vi "Test Func Mask.vi"() -> ()   [LabVIEW 2016]
uses:
  <vilib>/measure/mamon.llb/Create Continuous Mask using Formula.vi
  <vilib>/measure/mamon.llb/Limit Testing Time.vi
  <vilib>/measure/NI_MAPro.lvlib
  <vilib>/measure/NI_MABase.lvlib
panel:
  out "Limit":cluster{"x0":dbl, "dx":dbl, "Y":dbl[]} {"Y" format="%.2p"; "dx" format="%.2p"; "x0" format="%.2p"}
  out "Waveform Graph 3":waveform(dbl)[](graph)
  in  "stop":bool
  out "Waveform Graph":waveform(dbl)(graph)
  in  "signal type":T1(ring)
  in  "frequency":dbl=10.0 format="%0.2p"
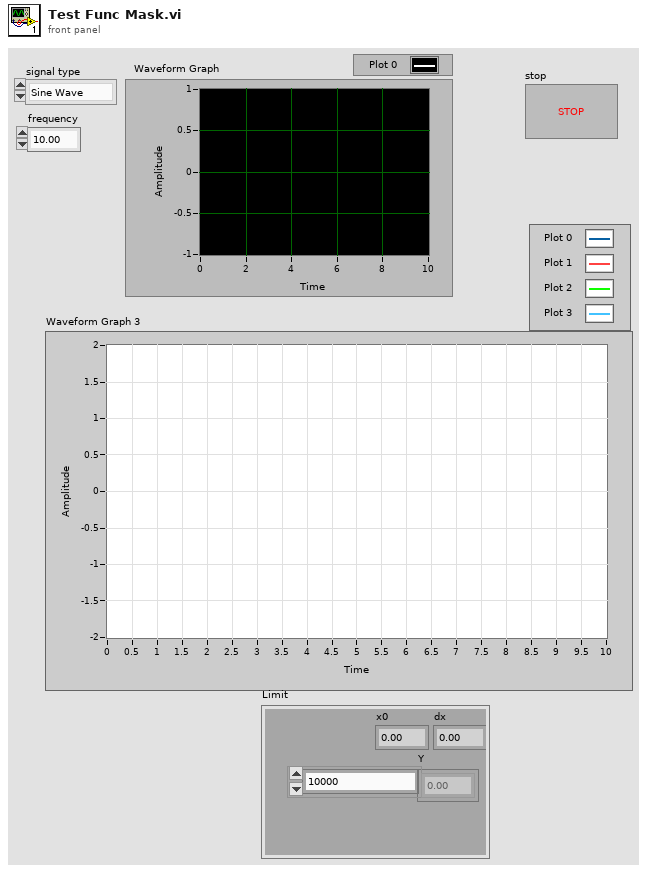
[diagram p1: front panel]
types:
  T1 = enum16{"Sine Wave", "Triangle Wave", "Square Wave", "Sawtooth Wave"}
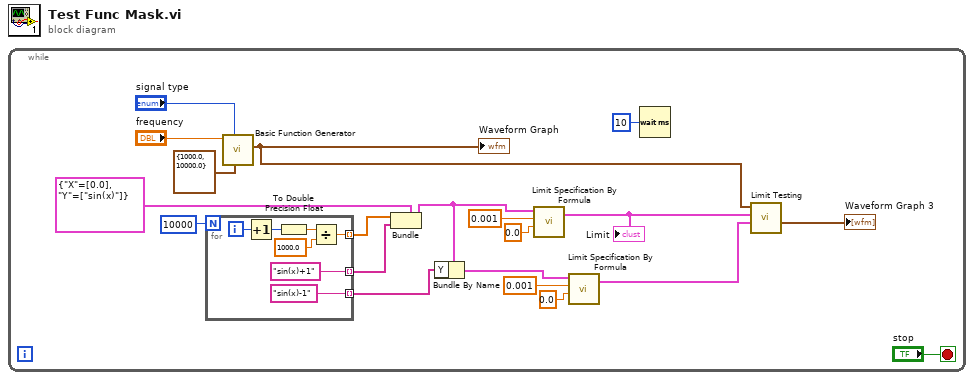
[diagram p0: block diagram]
diagram:
  n1 = while {
    stop <- "stop" stop-if-true
    n2 = for {
      N: 10000 -> [_]
      tunnel: [w27] -> w13 mode=indexing
      tunnel: ["sin(x)+1" ("String")] -> w11 mode=indexing
      tunnel: ["sin(x)-1" ("String")] -> w2 mode=indexing
      i -> [w24]
      n3 = Increment(x=w24) -> (x+1=w26:i32)
      n4 = To Double Precision Float(number=w26) -> (double precision float=w23:dbl)
      n5 = Divide(x=w23, y=1000.0) -> (x/y=w27:dbl)
    }
    n6 = call <vilib>:"Basic Function Generator.vi"("sampling info"=cluster{"Fs":dbl, "#s":dbl} {"Fs"=1000.0, "#s"=10000.0}, "signal type"="signal type", "frequency"="frequency") -> ("signal out"=w8:waveform(dbl))  [unwired: 6 in, 2 out]
    "Waveform Graph" <- w8
    n7 = Bundle(cluster=cluster{"X":dbl[], "Y":string[]} {"X"=[0.0], "Y"=["sin(x)"]} ("Specification Cluster"), "X"=w13, "Y"=w11) -> (w4:cluster{"X":dbl[], "Y":string[]})
    n8 = Bundle By Name(cluster=w4, "Y"=w2) -> (w3:cluster{"X":dbl[], "Y":string[]})
    n9 = call-poly <vilib>:"Limit Specification By Formula.vi"("Specification Cluster"=w4, "dx"=0.001, "x0"=0.0) -> ("Limit"=w9:cluster{"x0":dbl, "dx":dbl, "Y":dbl[]})  [unwired: 2 in, 1 out]
    "Limit" <- w9
    n10 = call-poly <vilib>:"Limit Specification By Formula.vi"("Specification Cluster"=w3, "dx"=0.001, "x0"=0.0) -> ("Limit"=w5:cluster{"x0":dbl, "dx":dbl, "Y":dbl[]})  [unwired: 2 in, 1 out]
    n11 = Wait (ms)(milliseconds to wait=u32 10) -> ()  [unwired: 1 out]
    n12 = call-poly <vilib>:"Limit Testing.vi"("lower limit"=w5, "upper limit"=w9, "signal in"=w8) -> ("output values"=→"Waveform Graph 3":waveform(dbl)[])  [unwired: 3 in, 5 out]
  }
